vi "2DGaussianRotationModel.vi"(3 "output control":T1, 4 "data":T2, 5 "X":dbl[](array[numeric]), 6 "a":dbl[](array[numeric])) -> (0 "error out":errorcluster, 1 "f'(X,a)":dbl[][](array[numeric]), 2 "f(X,a)":dbl[](array[numeric]))   [LabVIEW 2015]
doc: "This template is the starting point for creating a model function to be passed to the Nonlinear Curve Fit.vi."
uses:
  <vilib>/gmath/NumericalOptimization/objective function data.ctl
  <vilib>/gmath/NumericalOptimization/LM_output select.ctl
  <vilib>/Analysis/baseanly.llb/A x Vector.vi
  <vilib>/Analysis/Matrix/Numeric/Conversions/Array To Matrix - RA2.vi
  <vilib>/Analysis/NI_AALBase.lvlib
  <vilib>/Analysis/Matrix/NI_Matrix.lvlib
  <vilib>/gmath/NI_Gmath.lvlib
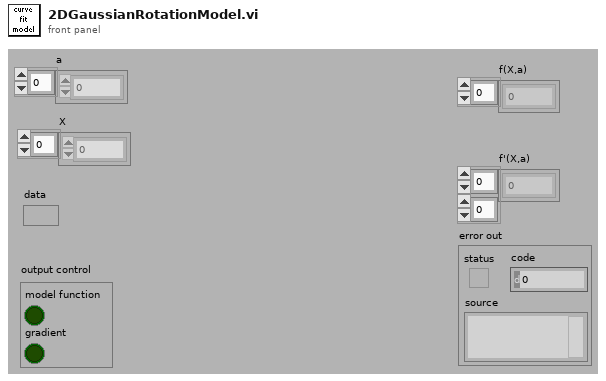
[diagram p1: front panel]
types:
  T1 = typedef "NI_Gmath.lvlib/LM_output select.ctl" = cluster{"model function":bool, "gradient":bool}
  T2 = typedef "NI_Gmath.lvlib/objective function data.ctl" = variant
  T3 = typedef "NI_Matrix.lvlib/RealMatrix.ctl" = dbl[][]
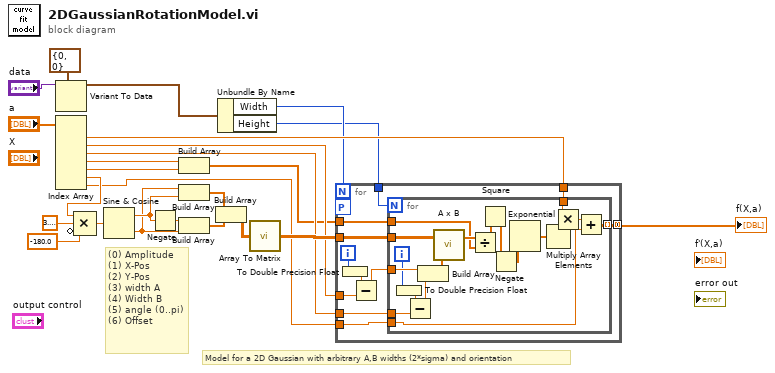
[diagram p0: block diagram]
diagram:
  # "Model for a 2D Gaussian with arbitrary A,B widths (2*sigma) and orientation"
  # "(0) Amplitude\n(1) X-Pos\n(2) Y-Pos\n(3) width A\n(4) Width B\n(5) angle (0..pi)\n(6) Offset"
  n1 = Variant To Data(type=cluster{"Width":i32, "Height":i32} {"Width"=0, "Height"=0} ("Plot Area:Size"), Variant="data") -> (data=w14:cluster{"Width":i32, "Height":i32})  [unwired: 1 in, 1 out]
  n2 = Index Array(array="a") -> (element #1=w18:dbl, element #2=w9:dbl, element #3=w8:dbl, element #4=w17:dbl, element #5=w16:dbl, element #6=w3:dbl, element #7=w2:dbl)  [unwired: 7 in]
  n3 = Compound Arithmetic op=MULTIPLY(w3, 3.141592653589793, invert -180.0 ("value")) -> (w7:dbl)
  n4 = Sine & Cosine(0:w7) -> (1:w24:dbl, 2:w23:dbl)
  n5 = Negate(x=w24) -> (-x=w25:dbl)
  n6 = Build Array(w17, w16) -> (w4:dbl[])
  n7 = Build Array(w23, w24) -> (w22:dbl[])
  n8 = Build Array(w25, w23) -> (w21:dbl[])
  n9 = Build Array(w22, w21) -> (w20:dbl[][])
  n10 = Unbundle By Name(w14) -> ("Width"=w11:i32, "Height"=w10:i32)
  n11 = call-poly <vilib>:"Array To Matrix.vi"("Real 2D Array"=w20) -> ("Real Matrix"=w19:T3)
  n12 = for {
    N: w11 -> [_]
    tunnel: w19 -> [w36]
    tunnel: w4 -> [w35]
    tunnel: [w34] -> w1 mode=concatenating
    tunnel: w18 -> [w33]
    tunnel: w10 -> [w32]
    tunnel: w9 -> [w29]
    tunnel: w8 -> [w27]
    workers-P: _ -> [_]
    tunnel: w2 -> [w26]
    i -> [w31]
    n13 = To Double Precision Float(number=w31) -> (double precision float=w30:dbl)
    n14 = Subtract(x=w30, y=w29) -> (x-y=w28:dbl)
    n15 = for {
      N: w32 -> [_]
      tunnel: w28 -> [w54]
      tunnel: w36 -> [w52]
      tunnel: w35 -> [w50]
      tunnel: [w38] -> w34 mode=indexing
      tunnel: w33 -> [w46]
      tunnel: w27 -> [w43]
      tunnel: w26 -> [w37]
      i -> [w45]
      n16 = To Double Precision Float(number=w45) -> (double precision float=w44:dbl)
      n17 = Subtract(x=w44, y=w43) -> (x-y=w42:dbl)
      n18 = Build Array(w54, w42) -> (w53:dbl[])
      n19 = call-poly <vilib>:"A x B.vi"("Vector"=w53, "A"=w52) -> ("A x Vector"=w51:dbl[])  [unwired: 1 out]
      n20 = Divide(x=w51, y=w50) -> (x/y=w41:dbl[])
      n21 = Square(x=w41) -> (x^2=w40:dbl[])
      n22 = Negate(x=w40) -> (-x=w39:dbl[])
      n23 = Exponential(1:w39) -> (0:w49:dbl[])
      n24 = Multiply Array Elements(1:w49) -> (0:w48:dbl)
      n25 = Multiply(x=w46, y=w48) -> (x*y=w47:dbl)
      n26 = Add(x=w47, y=w37) -> (x+y=w38:dbl)
    }
  }
  "f(X,a)" <- w1
